vi "Initialize.vi"(8 "Error in":errorcluster, 11 "VISA resource name":refnum<visa-resource-name>) -> (0 "Error out":errorcluster, 3 "VISA resource name out":refnum<visa-resource-name>)   [LabVIEW 2020, in "plugin_flodx_ph_probe.lvlib" / "mock_driver.lvlib"]
doc: "Simulates initializing the connection."
uses:
  mock_driver.lvlib
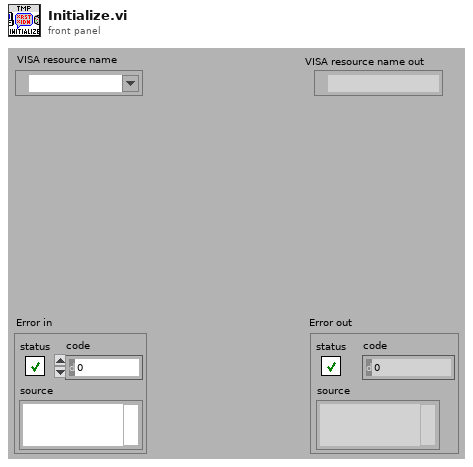
[diagram p1: front panel]
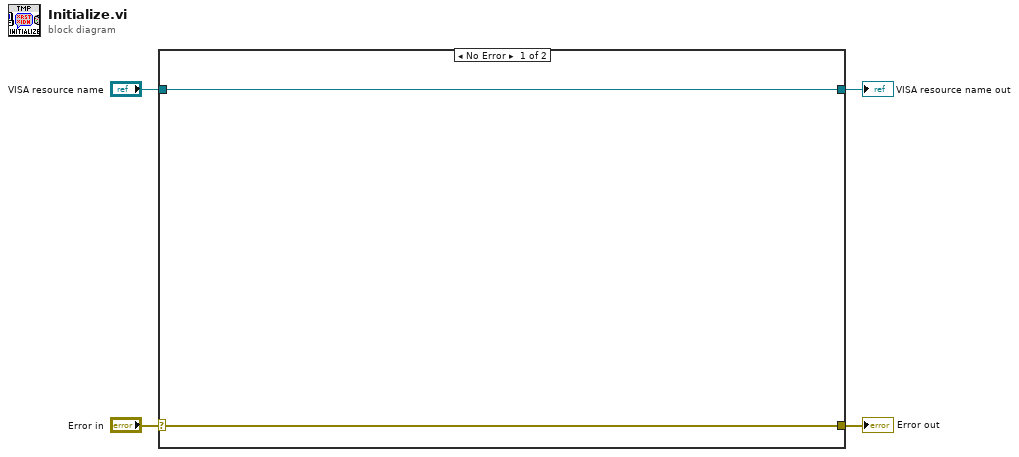
[diagram p0: block diagram]
diagram:
  n1 = case shown="No Error" "Error in" {
    selector: "Error in" -> [w6 w8]
    tunnel: "VISA resource name" -> [w5 w7]
    tunnel: [w6 w8] -> w3
    tunnel: [w5 w7] -> w1
    frame No Error {
    }
    frame Error {
    }
  }
  "VISA resource name out" <- w1
  "Error out" <- w3
